vi "DAQ@MergeWaveForm__Parameter.vi"(1 "ParamterIn":string) -> (0 "ParamterOut":string)   [LabVIEW 2020]
panel:
  out "WaveFormNameList":string[](array[string])
  in  "WaveForms":string(combo)
  in  "WaveFormName":string(combo)
  in  "Confirm":bool
  # "DAQ@MergeWaveForm $WaveForm,$WaveForm1,$WaveForm2(,$WaveForm3..)"
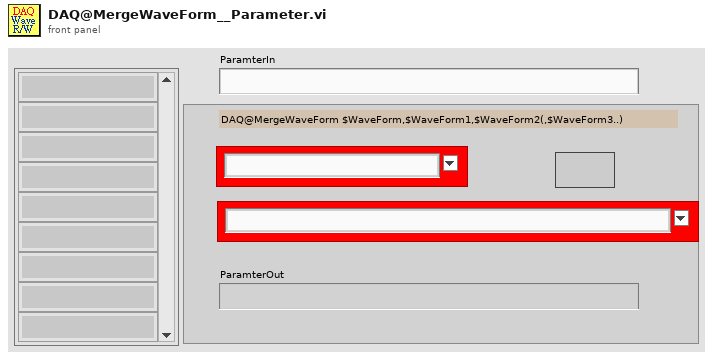
[diagram p1: front panel]
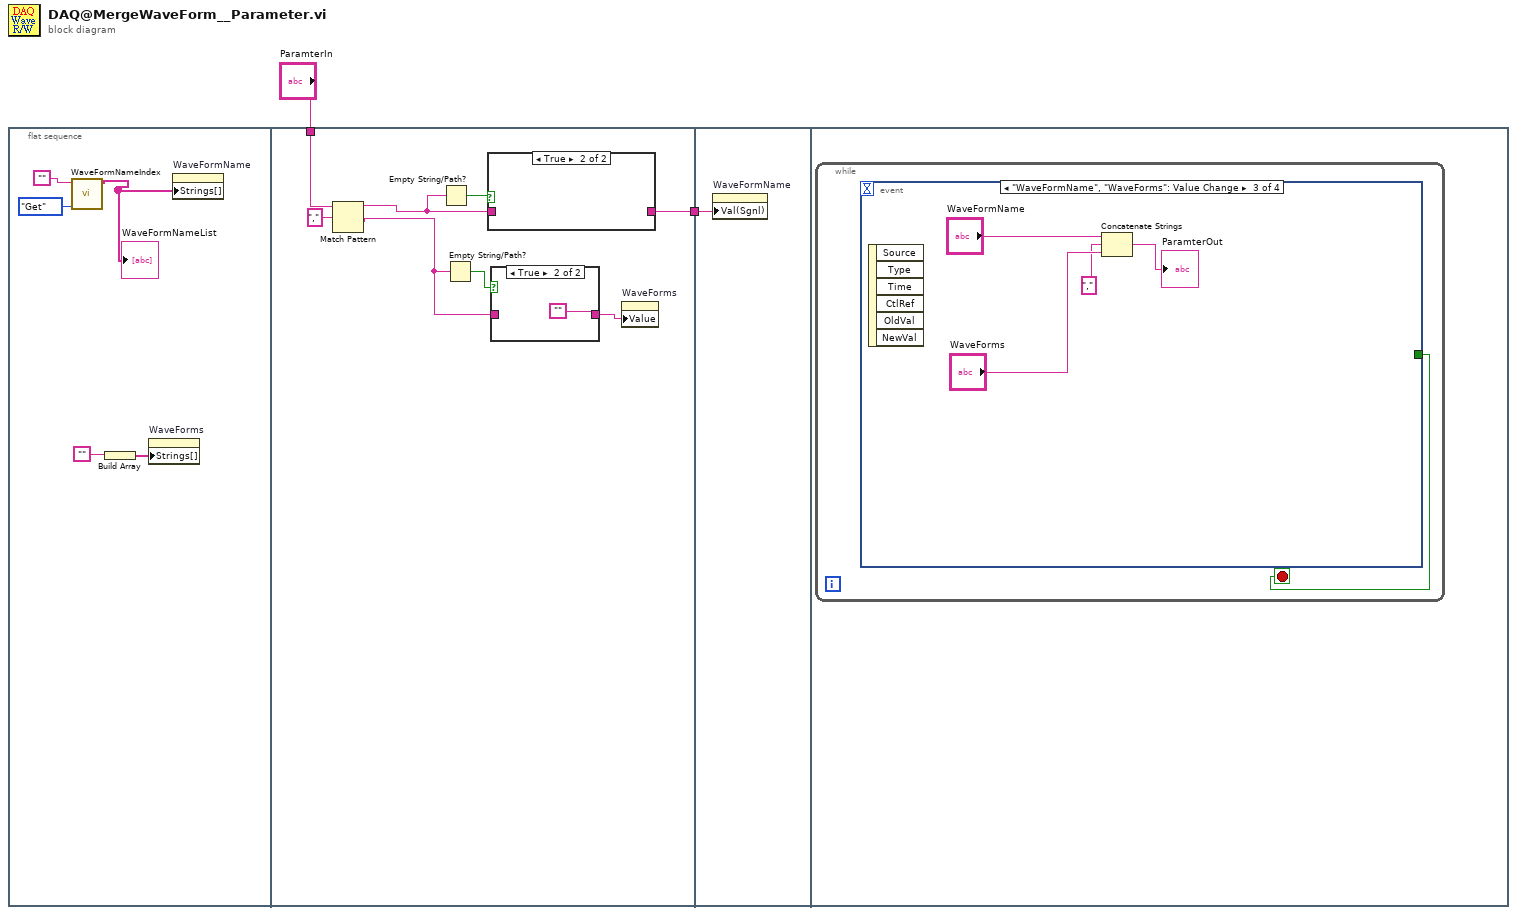
[diagram p0: block diagram]
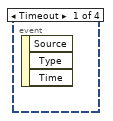
[diagram p4: hidden frame]
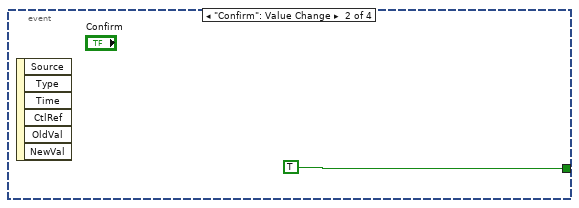
[diagram p5: hidden frame]
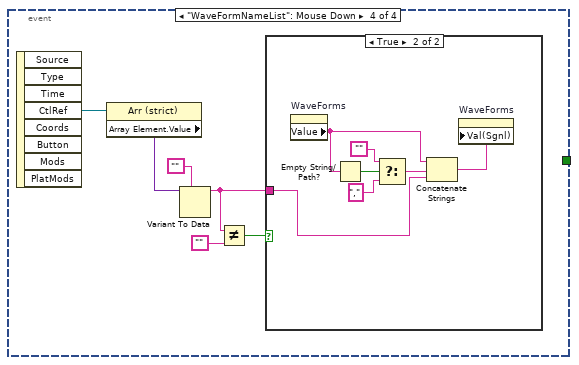
[diagram p6: hidden frame]
diagram:
  n1 = flat-sequence {
    tunnel: "ParamterIn" -> [w11]
    tunnel: [w12] -> w1
    tunnel: w1 -> [w19]
    frame #0 {
      n2 = call "WaveFormNameIndex.vi"("OP"=enum16{"Get", "Update", "Init", "GetSPS"}."Get", "WaveFormName"="") -> ("WaveFormNameList"=w5:string[])  [unwired: 6 in, 3 out]
      "WaveFormNameList" <- w5
      n3 = Build Array("") -> (w3:string[])
      n4 = property on="WaveForms" class="CmbBox"("Strings[]"=w3) -> ()  [unwired: 2 in, 2 out]
      n5 = property on="WaveFormName" class="CmbBox"("Strings[]"=w5) -> ()  [unwired: 2 in, 2 out]
    }
    frame #1 {
      n6 = Match Pattern(string=w11, regular expression=",") -> (before substring=w9:string, after substring=w8:string)  [unwired: 1 in, 2 out]
      n7 = Empty String/Path?(string/path=w9) -> (empty?=w15:bool)
      n8 = Empty String/Path?(string/path=w8) -> (empty?=w14:bool)
      n9 = case shown="True" w15 {
        tunnel: w9 -> [w18 _]
        tunnel: [w18 _] -> w12
        frame False {
        }
        frame True {
        }
      }
      n10 = case shown="True" w14 {
        tunnel: [w16 ""] -> w13
        tunnel: w8 -> [w16 _]
        frame False {
        }
        frame True {
        }
      }
      n11 = property on="WaveForms" class="CmbBox"("Value"=w13) -> ()  [unwired: 2 in, 2 out]
    }
    frame #2 {
      n12 = property on="WaveFormName" class="CmbBox"("Val(Sgnl)"=w19) -> ()  [unwired: 2 in, 2 out]
    }
    frame #3 {
      n13 = while {
        stop <- w20 stop-if-true
        n14 = event shown="[2] \"WaveFormName\", \"WaveForms\": Value Change" {
          selector: _ -> [_ _ _ _]
          dyn-events: _ -> [_ _ _ _]
          timeout: _ -> [_ _ _ _]
          tunnel: [_ TRUE _ _] -> w20
          event Timeout {
            n15 = event-data() -> ()  [unwired: 1 in, 3 out]
          }
          event "Confirm": Value Change {
            n16 = event-data() -> ()  [unwired: 1 in, 6 out]
          }
          event "WaveFormName", "WaveForms": Value Change {
            n17 = event-data() -> ()  [unwired: 1 in, 6 out]
            n18 = Concatenate Strings("WaveFormName", ",", "WaveForms") -> (→"ParamterOut":string)
          }
          event "WaveFormNameList": Mouse Down {
            n19 = event-data() -> ("CtlRef"=w31:refnum<vi>)  [unwired: 1 in, 7 out]
            n20 = property class="Arr (strict)"(reference=w31) -> ("Array Element.Value"=w28:variant)  [unwired: 1 in, 2 out]
            n21 = Variant To Data(type="", Variant=w28) -> (data=w26:string)  [unwired: 1 in, 1 out]
            n22 = Not Equal?(x=w26, y="") -> (x != y?=w27:bool)
            n23 = case shown="True" w27 {
              tunnel: w26 -> [_ w34]
              frame False {
              }
              frame True {
                n24 = property on="WaveForms" class="CmbBox"() -> ("Value"=w33:string)  [unwired: 2 in, 2 out]
                n25 = Empty String/Path?(string/path=w33) -> (empty?=w38:bool)
                n26 = Select(t="", s=w38, f=",") -> (s? t:f=w35:string)
                n27 = Concatenate Strings(w33, w35, w34) -> (w32:string)
                n28 = property on="WaveForms" class="CmbBox"("Val(Sgnl)"=w32) -> ()  [unwired: 2 in, 2 out]
              }
            }
          }
        }
      }
    }
  }
